vi "Calibration Zone Checking .vi"(8 "error in (no error)":errorcluster, 9 "Impedance Z (10m)":dbl=0.01 min=0.01 max=100000000.0 format="%^.2e", 10 "Frequency (20)":dbl=20.0 min=20.0 max=1000000.0 format="%.2f", 11 "VISA resource name":refnum<visa-resource-name>) -> (0 "error out":errorcluster, 2 "Zone":i16, 3 "VISA resource name out":refnum<visa-resource-name>)   [LabVIEW 2015, in "Agilent 428X Series.lvlib"]
doc: "This control determine which zone of calibration accuracy to be used. The zone is divided as follows:\n\n---------------------------------------------------------------------------\n 9 8\n---------------------------------------------------------------------------\n 8\n---------------------------------------------------------------------------\n 4 5 6 7 ---------------------------------------------------------------------------\n 0 1 2 3\n---------------------------------------------------------------------------\n\nDisclaimer: All accuracy calculation VI's are not part of the original \n driver. They are provided for supplementry purpose only.\n If user desires very high accuracy data, please do or \n check the calculation seperately."
uses:
  Agilent 428X Series.lvlib
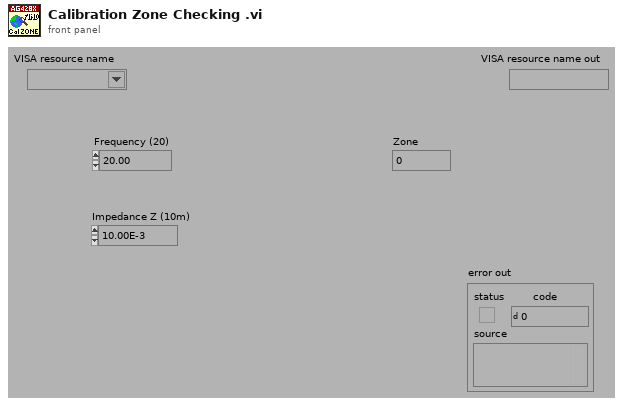
[diagram p1: front panel]
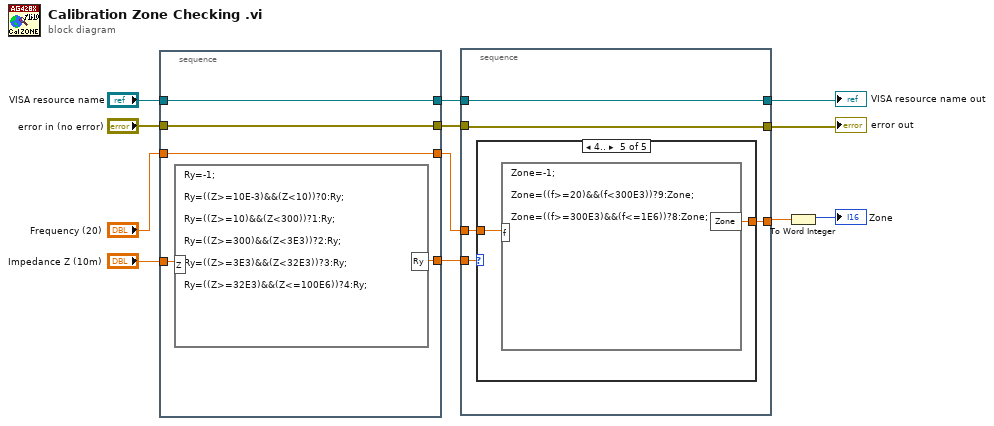
[diagram p0: block diagram]
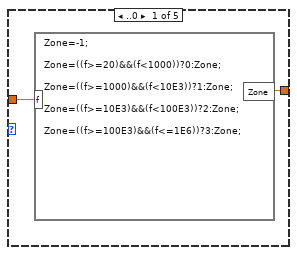
[diagram p2: hidden frame]
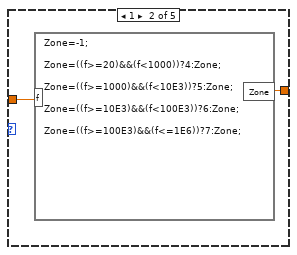
[diagram p3: hidden frame]
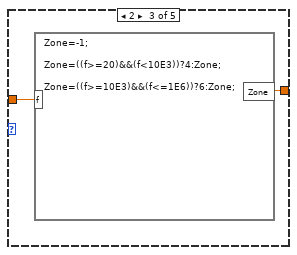
[diagram p4: hidden frame]
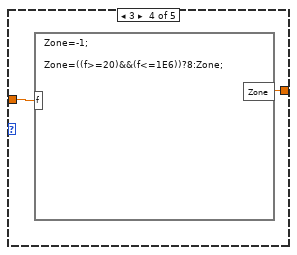
[diagram p5: hidden frame]
diagram:
  n1 = stacked-sequence {
    tunnel: "VISA resource name" -> [w17]
    tunnel: [w17] -> w11
    tunnel: [w14] -> w9
    tunnel: "Impedance Z (10m)" -> [w16]
    tunnel: [w15] -> w6
    tunnel: "error in (no error)" -> [w14]
    tunnel: "Frequency (20)" -> [w13]
    tunnel: [w13] -> w3
    frame #0 {
      n2 = formula code="Ry=-1;\n\nRy=((Z>=10E-3)&&(Z<10))?0:Ry;\n\nRy=((Z>=10)&&(Z<300))?1:Ry;\n\nRy=((Z>=300)&&(Z<3E3))?2:Ry;\n\nRy=((Z>=3E3)&&(Z<32E3))?3:Ry;\n\nRy=((Z>=32E3)&&(Z<=100E6))?4:Ry;"("Z"=w16) -> ("Ry"=w15:dbl)
    }
  }
  n3 = stacked-sequence {
    tunnel: w11 -> [w22]
    tunnel: [w22] -> w10
    tunnel: w9 -> [w21]
    tunnel: [w21] -> w8
    tunnel: w6 -> [w20]
    tunnel: [w19] -> w1
    tunnel: w3 -> [w18]
    frame #0 {
      n4 = case shown="4.." w20 {
        tunnel: [w24 w26 w28 w30 w32] -> w19
        tunnel: w18 -> [w23 w25 w27 w29 w31]
        frame ..0 {
          n5 = formula code="Zone=-1;\n\nZone=((f>=20)&&(f<1000))?0:Zone;\n\nZone=((f>=1000)&&(f<10E3))?1:Zone;\n\nZone=((f>=10E3)&&(f<100E3))?2:Zone;\n\nZone=((f>=100E3)&&(f<=1E6))?3:Zone;"("f"=w23) -> ("Zone"=w24:dbl)
        }
        frame 1 {
          n6 = formula code="Zone=-1;\n\nZone=((f>=20)&&(f<1000))?4:Zone;\n\nZone=((f>=1000)&&(f<10E3))?5:Zone;\n\nZone=((f>=10E3)&&(f<100E3))?6:Zone;\n\nZone=((f>=100E3)&&(f<=1E6))?7:Zone;"("f"=w25) -> ("Zone"=w26:dbl)
        }
        frame 2 {
          n7 = formula code="Zone=-1;\n\nZone=((f>=20)&&(f<10E3))?4:Zone;\n\nZone=((f>=10E3)&&(f<=1E6))?6:Zone;"("f"=w27) -> ("Zone"=w28:dbl)
        }
        frame 3 {
          n8 = formula code="Zone=-1;\n\nZone=((f>=20)&&(f<=1E6))?8:Zone;"("f"=w29) -> ("Zone"=w30:dbl)
        }
        frame 4.. {
          n9 = formula code="Zone=-1;\n\nZone=((f>=20)&&(f<300E3))?9:Zone;\n\nZone=((f>=300E3)&&(f<=1E6))?8:Zone;"("f"=w31) -> ("Zone"=w32:dbl)
        }
      }
    }
  }
  "VISA resource name out" <- w10
  "error out" <- w8
  n10 = To Word Integer(number=w1) -> (16bit integer=→"Zone":i16)
